vi "ConfigParams - Parse - UnitData.vi"(8 "error in (no error)":errorcluster, 11 "Ethernet in":refnum<class "ENET_BS1201.lvclass">) -> (0 "error out":errorcluster, 1 "Calibration Date":string, 2 "SerialNumber":string, 3 "Ethernet out":refnum<class "ENET_BS1201.lvclass">)   [LabVIEW 2021, in "BS120x Driver.lvlib" / "ENET_BS1201.lvclass"]
uses:
  ENET_BS1201.lvclass
panel:
  # "[UnitData]\nSerialNumber = \"abc123\"\nCalibration Date = \"DD/MM/YYYY\""
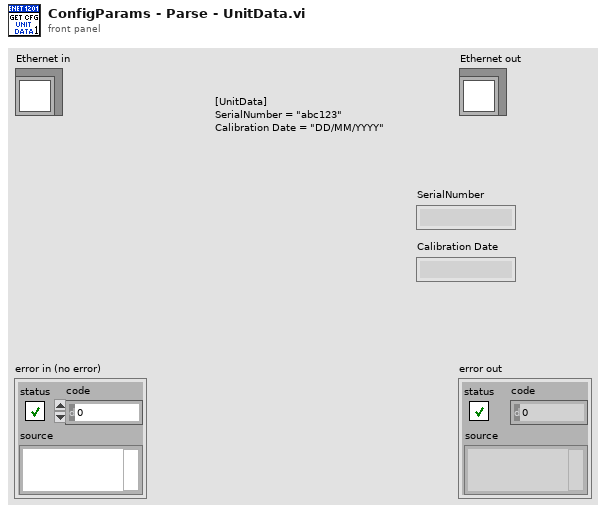
[diagram p1: front panel]
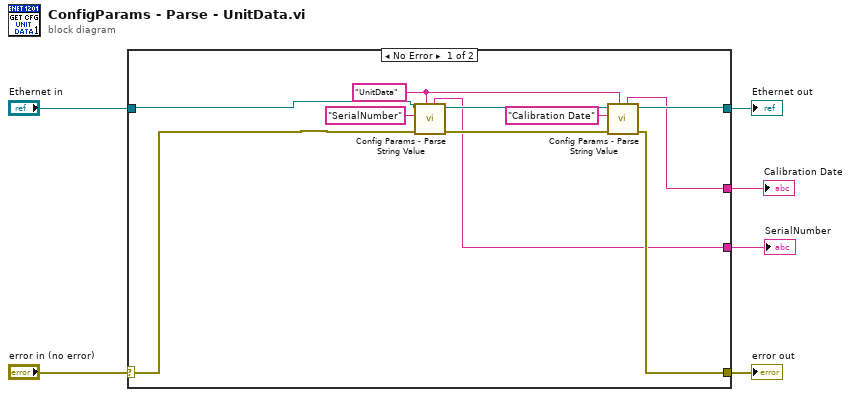
[diagram p0: block diagram]
diagram:
  n1 = case shown="No Error" "error in (no error)" {
    selector: "error in (no error)" -> [w10 w19]
    tunnel: [w11 w19] -> w5
    tunnel: [w12 w18] -> w3
    tunnel: "Ethernet in" -> [w9 w18]
    tunnel: [w8 _] -> w2
    tunnel: [w7 _] -> w1
    frame No Error {
      w14 = "UnitData" ("Section")
      n2 = call-dynamic "Config Params - Parse String Value.vi"("Section"=w14, "error in (no error)"=w10, "Key"="SerialNumber", "Ethernet in"=w9) -> ("error out"=w15:errorcluster, "Ethernet out"=w16:refnum<class "ENET_BS1201.lvclass">, "Value (str)"=w8:string)  [unwired: 1 in, 4 out]
      n3 = call-dynamic "Config Params - Parse String Value.vi"("Section"=w14, "error in (no error)"=w15, "Key"="Calibration Date", "Ethernet in"=w16) -> ("error out"=w11:errorcluster, "Ethernet out"=w12:refnum<class "ENET_BS1201.lvclass">, "Value (str)"=w7:string)  [unwired: 1 in, 4 out]
    }
    frame Error {
    }
  }
  "error out" <- w5
  "Ethernet out" <- w3
  "SerialNumber" <- w2
  "Calibration Date" <- w1
